vi "OPENDAQ_CONNECT.vi"(0 "VISA resourceINPUT":refnum<visa-resource-name>) -> (1 "connected to device":bool, 2 "VISA resource Salida":refnum<visa-resource-name>, 3 "error out":errorcluster, 4 "Gains":dbl[](array[numeric]), 5 "Offsets":dbl[](array[numeric]))   [LabVIEW 2011]
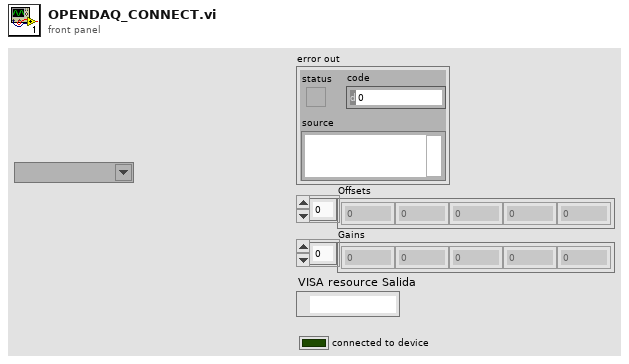
[diagram p1: front panel]
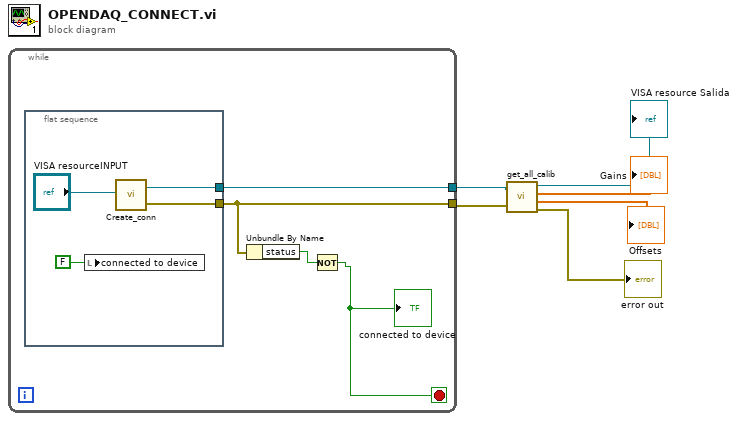
[diagram p0: block diagram]
diagram:
  n1 = while {
    tunnel: [w10] -> w6
    tunnel: [w9] -> w5
    stop <- w7 stop-if-true
    n2 = flat-sequence {
      tunnel: [w14] -> w10
      tunnel: [w13] -> w9
      frame #0 {
        n3 = local write "connected to device"(FALSE ("connected to device")) -> ()
        n4 = call "Create_conn.vi"("VISA resourceINPUT"="VISA resourceINPUT") -> ("error out"=w13:errorcluster, "VISA resource name out"=w14:refnum<visa-resource-name>)
      }
    }
    n5 = Unbundle By Name "Unbundle By Name"(w9) -> ("status"=w8:bool)
    n6 = Not(x=w8) -> (.not. x?=w7:bool)
    "connected to device" <- w7
  }
  n7 = call "get_all_calib.vi"("VISA resource name"=w6, "error in (no error)"=w5) -> ("VISA resource Salida"=→"VISA resource Salida":refnum<visa-resource-name>, "Gains"=→"Gains":dbl[], "Offsets"=→"Offsets":dbl[], "error out"=→"error out":errorcluster)
